vi "readData_SD.vi"(1 "how many points":i32) -> (0 "II channel seq":cluster{"BG":u16[], "Ie":u16[], "I0":u16[]}[](array[cluster]), 2 "I channel seq":cluster{"BG":u16[], "Ie":u16[], "I0":u16[]}[](array[cluster]))   [LabVIEW 2015]
panel:
  out "résultat début série":dbl[](array[numeric])
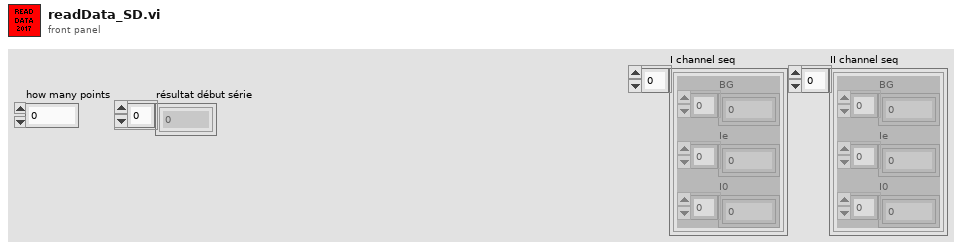
[diagram p1: front panel]
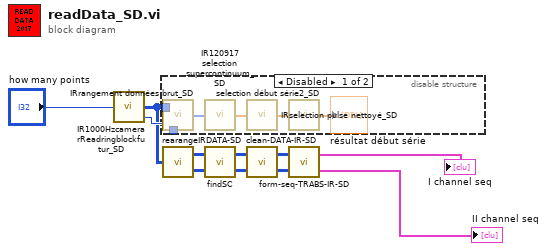
[diagram p0: block diagram]
diagram:
  n1 = call "IR1000HzcamerarReadringblockfutur_SD.vi"("Nombre d'acquisitions"="how many points") -> ("Data THz1000Hz"=w9:u32[][], "Nombre de spectres"=w10:i32)  [unwired: 1 out]
  n2 = disable-structure shown="Disabled" {
    disable-tunnel: w10 -> [w13 _]
    disable-tunnel: w9 -> [w12 _]
    frame Disabled {
      n3 = call "IRrangement données brut_SD.vi"("Nombre d'acquisition"=w13, "Brut camera"=w12) -> ("Data THz1000Hz"=w17:u16[])
      n4 = call "IR120917 selection supercontinuum_SD.vi"("DATA"=w17) -> ("résultat selec SC"=w15:dbl[])
      n5 = call "IRselection pulse nettoyé_SD.vi"("DATA"=w15) -> ("résultat pulse nettoyé"=w16:dbl[])
      n6 = call "selection début série2_SD.vi"("DATA"=w16) -> ("résultat début série"=→"résultat début série":dbl[])
    }
    frame Enabled {
    }
  }
  n7 = call "rearangeIRDATA-SD.vi"("Brut camera"=w9) -> ("I channel"=w6:u16[][], "II channel"=w5:u16[][])
  n8 = call "findSC.vi"("II channel"=w5, "I channel"=w6) -> ("II channel"=w3:u16[][], "I channel"=w4:u16[][])
  n9 = call "clean-DATA-IR-SD.vi"("II channel"=w3, "I channel"=w4) -> ("II channel cleaned"=w7:u16[][], "I channel cleaned"=w8:u16[][])
  n10 = call "form-seq-TRABS-IR-SD.vi"("II channel"=w7, "I channel"=w8) -> ("II channel seq"=→"II channel seq":cluster{"BG":u16[], "Ie":u16[], "I0":u16[]}[], "I channel seq"=→"I channel seq":cluster{"BG":u16[], "Ie":u16[], "I0":u16[]}[])
